vi "xps_panel_DO_perform_stage_action.vi"(8 "error in (no error)":errorcluster, 10 "xps_actions":T1, 11 "newport_xps_panel in":refnum<class "newport_xps_panel.lvclass">) -> (0 "error out":errorcluster, 3 "newport_xps_panel out":refnum<class "newport_xps_panel.lvclass">)   [LabVIEW 2015, in "newport_xps_panel.lvclass"]
uses:
  newport_xps_panel.lvclass
  xps_actions.ctl
  newport_xps/newport_xps.lvclass
  UI/panel_class/panel.lvclass
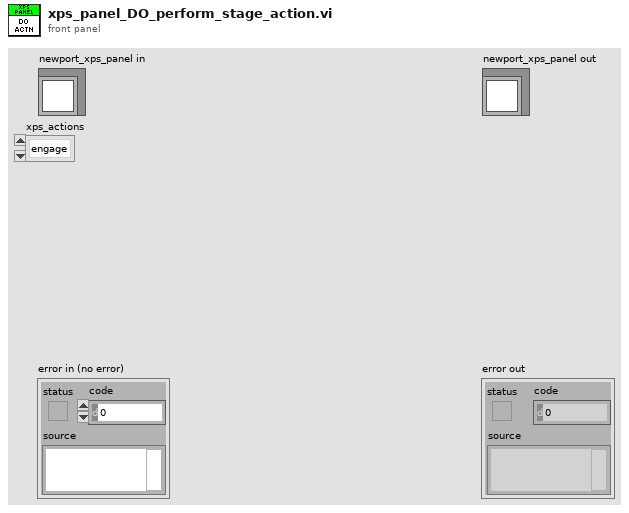
[diagram p1: front panel]
types:
  T1 = typedef "xps_actions.ctl" = enum16{"engage", "home", "kill"}
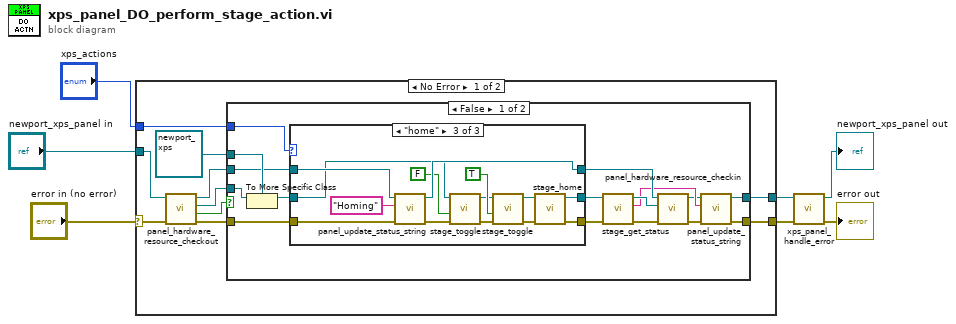
[diagram p0: block diagram]
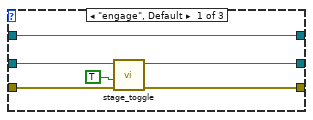
[diagram p2: hidden frame]
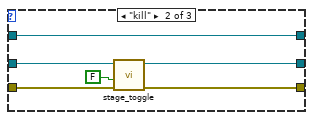
[diagram p3: hidden frame]
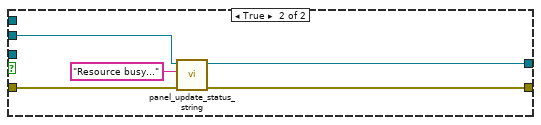
[diagram p4: hidden frame]
diagram:
  n1 = case shown="No Error" "error in (no error)" {
    selector: "error in (no error)" -> [w17 w66]
    tunnel: [w11 w66] -> w4
    tunnel: [w10 w65] -> w2
    tunnel: "newport_xps_panel in" -> [w16 w65]
    tunnel: "xps_actions" -> [w8 _]
    frame No Error {
      n2 = call "panel_hardware_resource_checkout.vi"("error in (no error)"=w17, "panel in"=w16) -> ("error out"=w12:errorcluster, "timed out?"=w15:bool, "hardware.lvclass"=w13:refnum<class "hardware.lvclass">, "panel out"=w14:refnum<class "newport_xps_panel.lvclass">)  [unwired: 6 in]
      n3 = case shown="False" w15 {
        tunnel: w14 -> [w28 w61]
        tunnel: w13 -> [w33 _]
        tunnel: w12 -> [w29 w64]
        tunnel: [w19 w63] -> w11
        tunnel: [w18 w60] -> w10
        tunnel: refnum<class "newport_xps.lvclass"> refnum ("newport_xps in") -> [w32 _]
        tunnel: w8 -> [w31 _]
        frame False {
          n4 = To More Specific Class(target class=w32, reference=w33) -> (specific class reference=w30:refnum<class "newport_xps.lvclass">)  [unwired: 1 in, 1 out]
          n5 = case shown="\"home\"" w31 {
            tunnel: w30 -> [w39 w45 w52]
            tunnel: w29 -> [w38 w44 w59]
            tunnel: w28 -> [w35 w41 w58]
            tunnel: [w35 w41 w57] -> w27
            tunnel: [w37 w43 w55] -> w25
            tunnel: [w36 w42 w54] -> w23
            frame "engage", Default {
              n6 = call-dynamic "stage_toggle.vi"("error in (no error)"=w38, "Engage?"=TRUE, "newport_xps in"=w39) -> ("error out"=w37:errorcluster, "newport_xps out"=w36:refnum<class "newport_xps.lvclass">)  [unwired: 7 in]
            }
            frame "kill" {
              n7 = call-dynamic "stage_toggle.vi"("error in (no error)"=w44, "Engage?"=FALSE, "newport_xps in"=w45) -> ("error out"=w43:errorcluster, "newport_xps out"=w42:refnum<class "newport_xps.lvclass">)  [unwired: 7 in]
            }
            frame "home" {
              n8 = call-dynamic "panel_update_status_string.vi"("error in (no error)"=w59, "String"="Homing", "newport_xps_panel in"=w58) -> ("error out"=w46:errorcluster, "newport_xps_panel out"=w57:refnum<class "newport_xps_panel.lvclass">)  [unwired: 7 in]
              n9 = call-dynamic "stage_toggle.vi"("error in (no error)"=w46, "Engage?"=FALSE, "newport_xps in"=w52) -> ("error out"=w50:errorcluster, "newport_xps out"=w49:refnum<class "newport_xps.lvclass">)  [unwired: 7 in]
              n10 = call-dynamic "stage_toggle.vi"("error in (no error)"=w50, "Engage?"=TRUE, "newport_xps in"=w49) -> ("error out"=w47:errorcluster, "newport_xps out"=w48:refnum<class "newport_xps.lvclass">)  [unwired: 7 in]
              n11 = call-dynamic "stage_home.vi"("error in (no error)"=w47, "newport_xps in"=w48) -> ("error out"=w55:errorcluster, "newport_xps out"=w54:refnum<class "newport_xps.lvclass">)  [unwired: 8 in]
            }
          }
          n12 = call-dynamic "stage_get_status.vi"("error in (no error)"=w25, "newport_xps in"=w23) -> ("error out"=w20:errorcluster, "Status"=w22:string, "newport_xps out"=w24:refnum<class "newport_xps.lvclass">)  [unwired: 7 in]
          n13 = call "panel_hardware_resource_checkin.vi"("error in (no error)"=w20, "hardware.lvclass"=w24, "panel in"=w27) -> ("error out"=w26:errorcluster, "panel out"=w21:refnum<class "newport_xps_panel.lvclass">)  [unwired: 7 in]
          n14 = call-dynamic "panel_update_status_string.vi"("error in (no error)"=w26, "String"=w22, "newport_xps_panel in"=w21) -> ("error out"=w19:errorcluster, "newport_xps_panel out"=w18:refnum<class "newport_xps_panel.lvclass">)  [unwired: 7 in]
        }
        frame True {
          n15 = call-dynamic "panel_update_status_string.vi"("error in (no error)"=w64, "String"="Resource busy...", "newport_xps_panel in"=w61) -> ("error out"=w63:errorcluster, "newport_xps_panel out"=w60:refnum<class "newport_xps_panel.lvclass">)  [unwired: 7 in]
        }
      }
    }
    frame Error {
    }
  }
  n16 = call "xps_panel_handle_error.vi"("error in (no error)"=w4, "newport_xps_panel in"=w2) -> ("error out"=→"error out":errorcluster, "newport_xps_panel out"=→"newport_xps_panel out":refnum<class "newport_xps_panel.lvclass">)  [unwired: 8 in]
